vi "FirePneumatic.vi"   [LabVIEW 2013]
uses:
  State_Machine_Enum.ctl
  <vilib>/Rock Robotics/WPI/Solenoid/WPI_SolenoidValue.ctl
  RefnameEnum.ctl
  <vilib>/Rock Robotics/WPI/Solenoid/WPI_SolenoidSetEnum.vi
  Robot Global Data.vi
types:
  T1 = typedef "State_Machine_Enum.ctl" = enum16{"Idle", "Start", "Do", "Stop", "Init"}
  T2 = typedef "RefnameEnum.ctl" = enum16{"FireLauncher", "Climber", "Shield", "TankDrive", "DriveEncoderL", "DriveEncoderR", "LauncherMotorRPM", "LauncherEncoderAnalog", "LauncherEncoderRPM", "ShooterLS", "DriveAlignLSLeft", "DriveAlignLSRight", "ClimbingLS", "LauncherEncoderAngle", "LauncherMotorAngle", "Gamepad1", "Gamepad2", "Compressor", "ClimbWeightSol3", "ClimbWeightSol4"}
  T3 = typedef "WPI_SolenoidValue.ctl" = enum16{"Off", "On", "Forward", "Reverse"}
  T4 = typedef "WPI_SolenoidDevRef.ctl" = cluster{"DevStatus":errorcluster, "Solenoid Module":T5, "Forward Solenoid Channel":T6, "Reverse Solenoid Channel":T6}
  T5 = typedef "FPGA_TypedefSolenoidModule.ctl" = enum16{"Solenoid Module 1", "Solenoid Module 2"}
  T6 = typedef "WPI_SolenoidChannel.ctl" = enum8{"Solenoid 1", "Solenoid 2", "Solenoid 3", "Solenoid 4", "Solenoid 5", "Solenoid 6", "Solenoid 7", "Solenoid 8", "Invalid"}
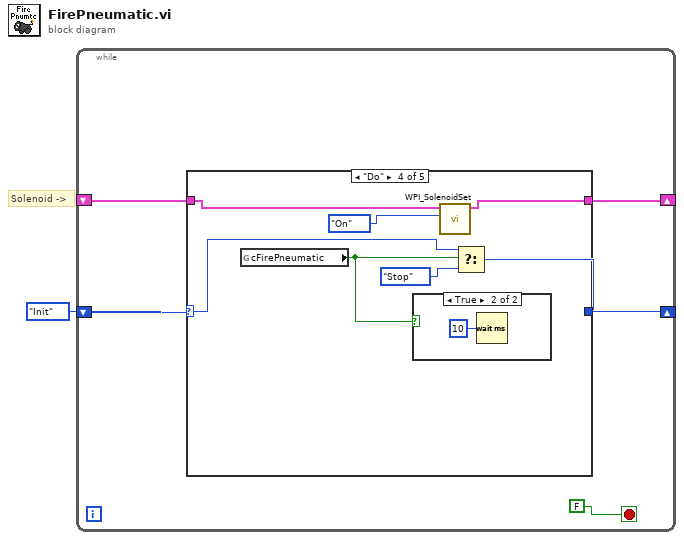
[diagram p0: block diagram]
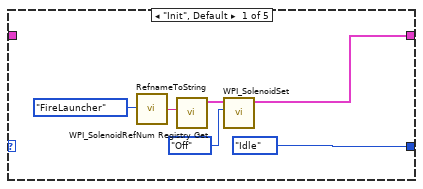
[diagram p2: hidden frame]
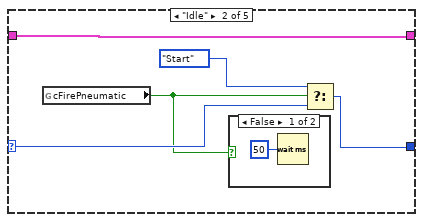
[diagram p3: hidden frame]
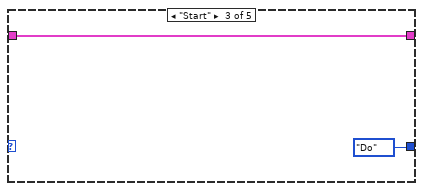
[diagram p5: hidden frame]
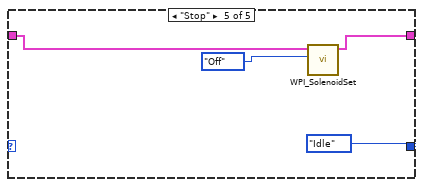
[diagram p7: hidden frame]
diagram:
  # "Solenoid ->"
  n1 = while {
    shift-right: [w3] -> _
    shift-left: State_Machine_Enum."Init" ("State") -> [w6]
    shift-right: [w5] -> _
    shift-left: _ -> [w4]
    stop <- FALSE stop-if-true
    n2 = case shown="\"Do\"" w6 {
      selector: w6 -> [_ w17 _ w21 _]
      tunnel: [w9 w13 w20 w25 w30] -> w5
      tunnel: w4 -> [_ w13 w20 w26 w31]
      tunnel: [State_Machine_Enum."Idle" ("State") w16 State_Machine_Enum."Do" ("State") w24 State_Machine_Enum."Idle" ("State")] -> w3
      frame "Init", Default {
        n3 = call "RefnameToString.vi"("Enum"=RefnameEnum."FireLauncher") -> ("Refname"=w7:string)
        n4 = call <vilib>:"WPI_SolenoidRefNum Registry Get.vi"("refnum name"=w7) -> ("SolenoidDevRef"=w10:T4)  [unwired: 9 in, 1 out]
        n5 = call-poly <vilib>:"WPI_SolenoidSet.vi"("Value"=WPI_SolenoidValue."Off", "SolenoidDevRef"=w10) -> ("SolenoidDevRef"=w9:T4)  [unwired: 1 in, 8 out]
      }
      frame "Idle" {
        n6 = global read "Robot Global Data.vi" "cFirePneumatic"() -> (w15:bool)
        n7 = case shown="False" w15 {
          frame False {
            n8 = Wait (ms)(milliseconds to wait=u32 50) -> ()  [unwired: 1 out]
          }
          frame True {
          }
        }
        n9 = Select(t=State_Machine_Enum."Start" ("State"), s=w15, f=w17) -> (s? t:f=w16:T1)
      }
      frame "Start" {
      }
      frame "Do" {
        n10 = global read "Robot Global Data.vi" "cFirePneumatic"() -> (w23:bool)
        n11 = case shown="True" w23 {
          frame False {
          }
          frame True {
            n12 = Wait (ms)(milliseconds to wait=u32 10) -> ()  [unwired: 1 out]
          }
        }
        n13 = call-poly <vilib>:"WPI_SolenoidSet.vi"("Value"=WPI_SolenoidValue."On", "SolenoidDevRef"=w26) -> ("SolenoidDevRef"=w25:T4)  [unwired: 1 in, 8 out]
        n14 = Select(t=w21, s=w23, f=State_Machine_Enum."Stop" ("State")) -> (s? t:f=w24:T1)
      }
      frame "Stop" {
        n15 = call-poly <vilib>:"WPI_SolenoidSet.vi"("Value"=WPI_SolenoidValue."Off", "SolenoidDevRef"=w31) -> ("SolenoidDevRef"=w30:T4)  [unwired: 1 in, 8 out]
      }
    }
  }
